vi "ALP1P.vi"() -> ()   [LabVIEW 2016]
doc: "This device can add or multiply two signals where the user if free to choose their amplitude, period and if is a sinusodial or square wave. The user can also add white noise and the amplitude of the noise. Also, the user can choose to filter those signal on a high pass and low pass filter each with 1st, 2nd or 3rd order for each a low pass or high pass filter. Lastly the user can change the update interval of the device.\n\nAlexis Lopez\nP350\nCSUSB Physics"
uses:
  typedefs/periodic signal control.ctl
  <vilib>/ptbypt/NI_PtbyPt.lvlib
panel:
  in  "Tab Control":enum32{"Signal generation", "Filtering"}(tab)
  in  "white noise":bool
  in  "white noise amplitude":dbl(slide)=0.2 scale=0.0..1.0
  in  "combo mode":bool=TRUE
  in  "Source B":T1={"source"=TRUE, "source type"=FALSE, "Amplitude"=1.0, "Period (steps)"=100.0} {"Amplitude" scale=0.0..1.0; "Period (steps)" scale=1.0..1000.0}
  in  "Source A":T1={"source"=TRUE, "source type"=FALSE, "Amplitude"=1.0, "Period (steps)"=10.0} {"Amplitude" scale=0.0..1.0; "Period (steps)" scale=1.0..1000.0}
  in  "HP Order":enum16{"3", "2", "1"}(ring)=enum."1"
  in  "LP Order":enum16{"1", "2", "3"}(ring)=enum."3"
  in  "High pass":bool
  in  "HP Corner Period":dbl(slide)=1.0 caption="High Pass Corner Period (steps)" scale=1.0..1000.0
  in  "LP Corner Period":dbl(slide)=57.2237 caption="Low Pass Corner Period (steps)" scale=1.0..1000.0
  in  "Low pass":bool=TRUE
  in  "update interval (ms)":u32(slide)=20 scale=1.0..1000.0
  in  "stop":bool
  out "Waveform Chart":cluster{"Signal out":dbl, "output":dbl}(graph)={"Signal out"=0.3632712640028559, "output"=-0.4254782850474608}
  # "Alexis Lopez\nPhysics 350\nCSUSB Physics"
  # "Signal Generation and Filtering"
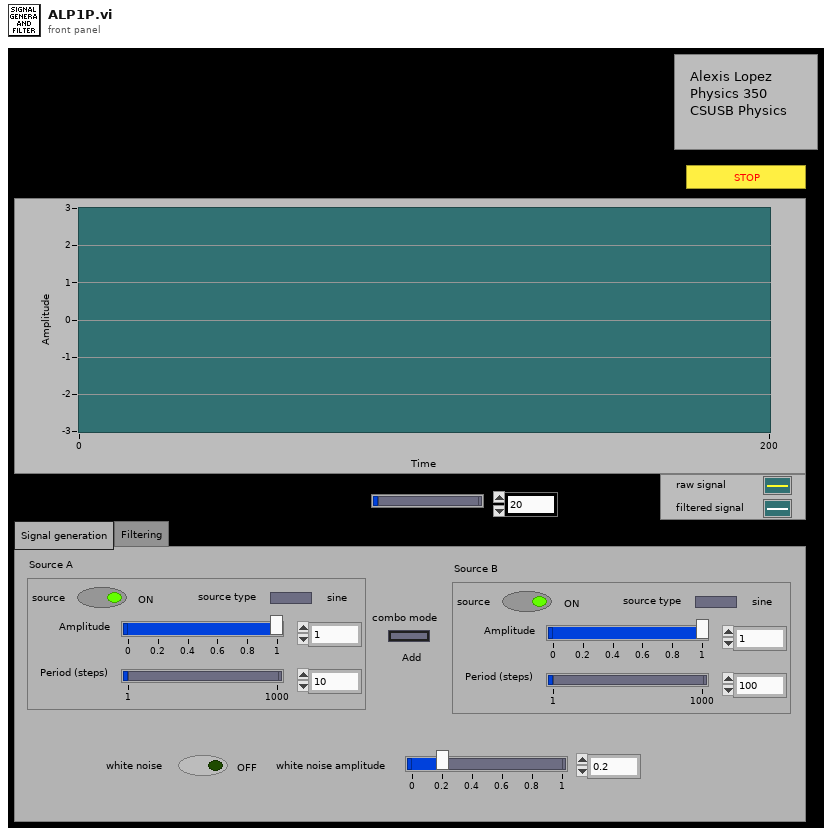
[diagram p1: front panel]
types:
  T1 = typedef "periodic signal control.ctl" = cluster{"source":bool, "source type":bool, "Amplitude":dbl, "Period (steps)":dbl}
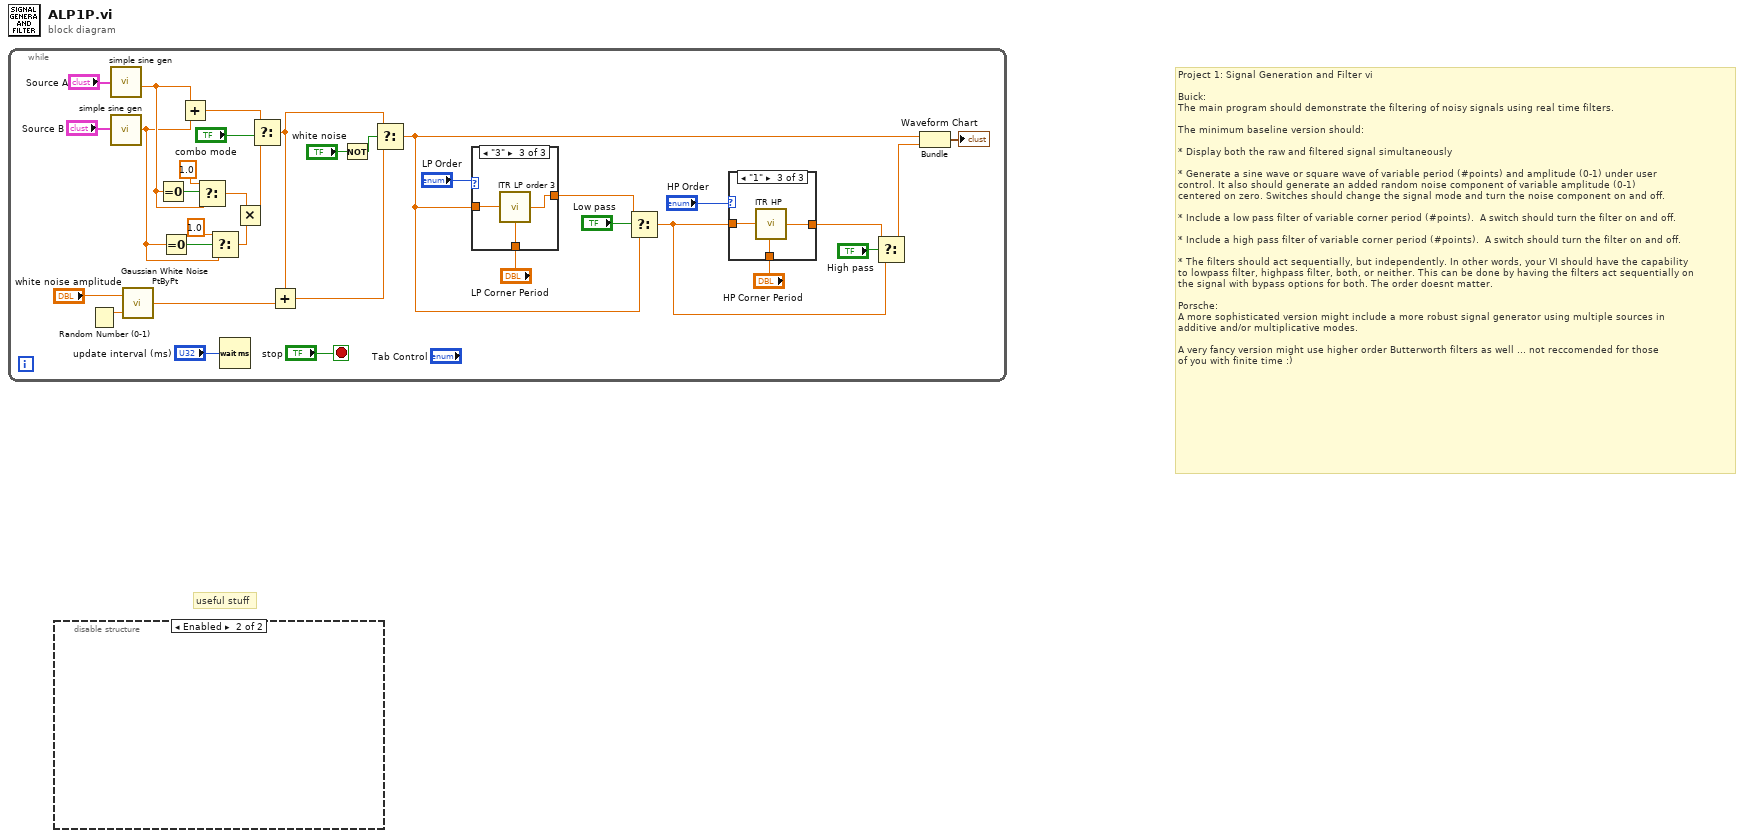
[diagram p0: block diagram]
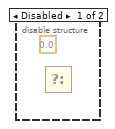
[diagram p2: hidden frame]
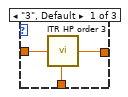
[diagram p3: hidden frame]
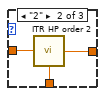
[diagram p4: hidden frame]
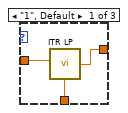
[diagram p5: hidden frame]
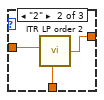
[diagram p6: hidden frame]
diagram:
  # "Project 1: Signal Generation and Filter vi\n\nBuick:\nThe main program should demonstrate the filtering of noisy signals using real time filters.\n\nThe minimum baseline version should:\n\n* Display both the raw and filtered signal simultaneously\n\n* Generate a sine wave or square wave of variable period (#points) and amplitude (0-1) under user\ncontrol. It also should generate an added random noise component of variable amplitude (0-1) \ncentered on zero. Switches should change the signal mode and turn the noise component on and off.\n\n* Include a low pass filter of variable corner period (#points).  A switch should turn the filter on and off.\n\n* Include a high pass filter of variable corner period (#points).  A switch should turn the filter on and off.\n\n* The filters should act sequentially, but independently. In other words, your VI should have the capability \nto lowpass filter, highpass filter, both, or neither. This can be done by having the filters act sequentially on\nthe signal with bypass options for both. The order doesnt matter.\n\nPorsche:\nA more sophisticated version might include a more robust signal generator using multiple sources in \nadditive and/or multiplicative modes.\n\nA very fancy version might use higher order Butterworth filters as well ... not reccomended for those\nof you with finite time :)"
  # "useful stuff"
  n1 = while {
    stop <- "stop" stop-if-true
    n2 = Random Number (0-1)() -> (number: 0 to 1=w17:dbl)
    n3 = call "simple sine gen.vi"("Source"="Source A") -> ("output"=w7:dbl)  [unwired: 14 in]
    n4 = call "simple sine gen.vi"("Source"="Source B") -> ("output"=w4:dbl)  [unwired: 14 in]
    n5 = call <vilib>:"Gaussian White Noise PtByPt.vi"("seed"=w17, "standard deviation"="white noise amplitude") -> ("Gaussian white noise"=w32:dbl)  [unwired: 1 in]
    n6 = Equal To 0?(x=w7) -> (x = 0?=w8:bool)
    n7 = Equal To 0?(x=w4) -> (x = 0?=w5:bool)
    n8 = Add(x=w7, y=w4) -> (x+y=w23:dbl)
    n9 = Select(t=1.0, s=w8, f=w7) -> (s? t:f=w6:dbl)
    n10 = Select(t=1.0, s=w5, f=w4) -> (s? t:f=w3:dbl)
    n11 = Wait (ms)(milliseconds to wait="update interval (ms)") -> ()  [unwired: 1 out]
    n12 = Multiply(x=w6, y=w3) -> (x*y=w22:dbl)
    n13 = Select(t=w23, s="combo mode", f=w22) -> (s? t:f=w21:dbl)
    n14 = Add(x=w21, y=w32) -> (x+y=w31:dbl)
    n15 = Not(x="white noise") -> (.not. x?=w26:bool)
    n16 = Select(t=w21, s=w26, f=w31) -> (s? t:f=w15:dbl)
    n17 = case shown="\"3\"" "LP Order" {
      tunnel: w15 -> [w46 w49 w52]
      tunnel: "LP Corner Period" -> [w45 w48 w51]
      tunnel: [w44 w47 w50] -> w13
      frame "1", Default {
        n18 = call "ITR LP.vi"("input"=w46, "corner period (steps)"=w45) -> ("output"=w44:dbl)  [unwired: 13 in]
      }
      frame "2" {
        n19 = call "ITR LP order 2.vi"("input"=w49, "corner period (steps)"=w48) -> ("output"=w47:dbl)  [unwired: 13 in]
      }
      frame "3" {
        n20 = call "ITR LP order 3.vi"("input"=w52, "corner period (steps)"=w51) -> ("output"=w50:dbl)  [unwired: 13 in]
      }
    }
    n21 = Select(t=w13, s="Low pass", f=w15) -> (s? t:f=w11:dbl)
    n22 = case shown="\"1\"" "HP Order" {
      tunnel: w11 -> [w35 w39 w43]
      tunnel: "HP Corner Period" -> [w37 w40 w42]
      tunnel: [w36 w38 w41] -> w9
      frame "3", Default {
        n23 = call "ITR HP order 3.vi"("input"=w35, "corner period (steps)"=w37) -> ("output"=w36:dbl)  [unwired: 13 in]
      }
      frame "2" {
        n24 = call "ITR HP order 2.vi"("input"=w39, "corner period (steps)"=w40) -> ("output"=w38:dbl)  [unwired: 13 in]
      }
      frame "1" {
        n25 = call "ITR HP.vi"("input"=w43, "corner period (steps)"=w42) -> ("output"=w41:dbl)  [unwired: 13 in]
      }
    }
    n26 = Select(t=w9, s="High pass", f=w11) -> (s? t:f=w28:dbl)
    n27 = Bundle(w15, "output"=w28) -> (→"Waveform Chart":cluster{dbl, "output":dbl})  [unwired: 1 in]
  }
  n28 = disable-structure shown="Enabled" {
    frame Disabled {
      (unwired) 0.0 ("f")
      n29 = Select() -> ()  [unwired: 3 in, 1 out]
    }
    frame Enabled {
    }
  }
